vi "Alignment Error.vi"() -> ()   [LabVIEW 2012]
panel:
  in  "Alignment Error":dbl
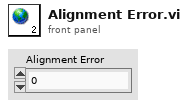
[diagram p1: front panel]
diagram:
